vi "close.vi"(8 "error in":errorcluster, 11 "Benchmark PID runtime in":refnum<class "Benchmark PID runtime.lvclass">) -> (0 "error out":errorcluster)   [LabVIEW 2018, in "Benchmark PID runtime.lvclass"]
doc: "Provides an interface for terminating a module instance. While this interface performs no operations, a child should close and deallocate any open references or memory."
uses:
  Benchmark PID runtime.lvclass
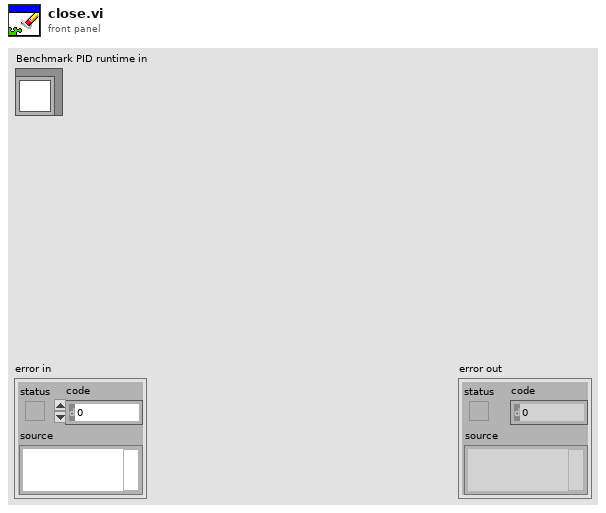
[diagram p1: front panel]
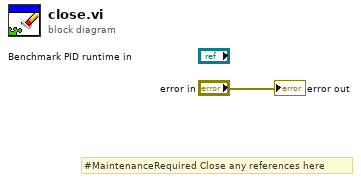
[diagram p0: block diagram]
diagram:
  # "#MaintenanceRequired Close any references here"
  "error out" <- "error in"
